vi "LV86_Convert to image.vi"(0 "Intensity Graph":u8[][](graph), 2 "Flip?":bool, 3 "Image In":T1 {"Dialogs" format="%.0b"}) -> (1 "Image Out":T1 {"Dialogs" format="%.0b"})   [LabVIEW 2024]
doc: "This VI converts a 2-dimensional array to an image. The image resolution is equal to the number of columns by the number of rows.\n\nModifier: \nFlip: If true, this will flip the image so that the image looks right in the Intensity graph (element 0,0 in a picture is the upper left corner but in a graph is in the lower left). Default is False."
uses:
  <userlib>/ImageProcessing/QTLIB_2595_LV86/QT_Image.ctl
panel:
  # "This VI converts a 2-dimensional array to an image.  \nThe image resolution is equal to the number of \ncolumns by the number of rows. \n\nModifier: \nFlip: If true, this will flip the image so that the image looks right in the Intensity graph (element 0,0  in a picture is the upper left corner but in a graph is in the lower left).  Default is False."
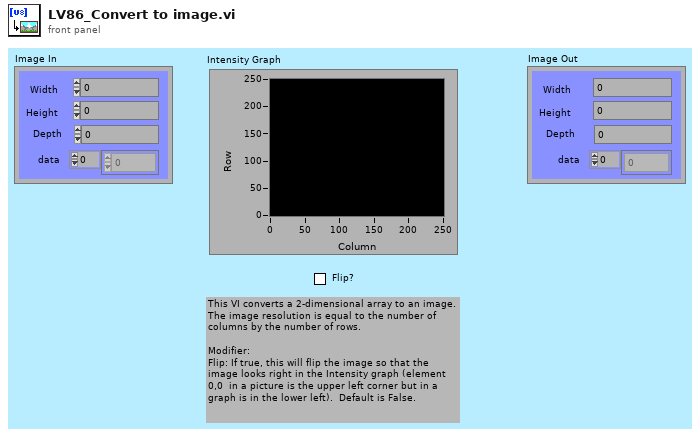
[diagram p1: front panel]
types:
  T1 = typedef "QT_Image.ctl" = cluster{"Width":i32, "Height":i32, "Depth":i32, "data":u8[], "Compressed data":u8[], "Color table":u32[], "Duration":i32, "Options":i32, "Timestamp":i32, "ID":i32, "Reserved":i32, "Dialogs":u32}
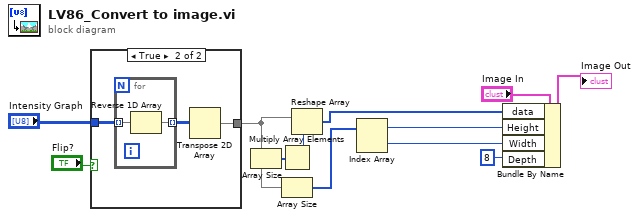
[diagram p0: block diagram]
diagram:
  n1 = case shown="True" "Flip?" {
    tunnel: "Intensity Graph" -> [w13 w16]
    tunnel: [w13 w14] -> w9
    frame False {
    }
    frame True {
      n2 = for {
        tunnel: w16 -> [w18] mode=indexing
        tunnel: [w17] -> w15 mode=indexing
        n3 = Reverse 1D Array(array=w18) -> (reversed array=w17:u8[])
      }
      n4 = Transpose 2D Array(2D array=w15) -> (transposed array=w14:u8[][])
    }
  }
  n5 = Array Size(array=w9) -> (size(s)=w10:i32[])
  n6 = Multiply Array Elements(1:w10) -> (0:w8:i32)
  n7 = Array Size(array=w9) -> (size(s)=w5:i32[])
  n8 = Reshape Array(w9, w8) -> (w4:u8[])
  n9 = Index Array(array=w5) -> (element #1=w3:i32, element #2=w2:i32)  [unwired: 2 in]
  n10 = Bundle By Name(cluster="Image In", "data"=w4, "Height"=w3, "Width"=w2, "Depth"=8) -> (→"Image Out":T1)
